vi "Receive Value Change Msg.vi"(8 "error in (no error)":errorcluster, 10 "ValueChangeMsg":refnum<class "ValueChangeMsg.lvclass">, 11 "MediatorBusMonitor In":refnum<class "MediatorBusMonitor.lvclass">) -> (0 "error out":errorcluster, 3 "MediatorBusMonitor Out":refnum<class "MediatorBusMonitor.lvclass">)   [LabVIEW 2015, in "Mediator.lvlib" / "MediatorBusMonitor.lvclass"]
doc: "<License>\nCopyright © 2017 Composed Systems, LLC | All rights reserved\nwww.composed.io\n\nAuthor: Ethan Stern <ethan.stern@composed.io>\n\nThis software is provided \"AS IS\" WITHOUT WARRANTIES, either express or implied, AND IS FOR EDUCATIONAL PURPOSES ONLY.\n</License>"
uses:
  MediatorBusMonitor.lvclass
  AutoRegistration/ActorAutoRegistration Messages/ValueChangeMsg/ValueChangeMsg.lvclass
  MediatorBusMonitor.lvclass/MediatorBusMonitor.ctl
  <vilib>/ActorFramework/Time-Delayed Send Message/Time-Delay Override Options.ctl
  MediatorBusMonitor Messages/Update Front Panel Msg/Update Front Panel Msg.lvclass
  <vilib>/ActorFramework/Actor/Actor.lvclass/Actor.ctl
  <vilib>/ActorFramework/Message Enqueuer/Message Enqueuer.lvclass/Message Enqueuer.ctl
  <vilib>/ActorFramework/Message Enqueuer/Init from Existing Queue.vi
  <vilib>/ActorFramework/Message Enqueuer/Message Enqueuer.lvclass
  Components/CurrentValueTable/CurrentValueTable.lvclass
  <vilib>/ActorFramework/Actor/Actor.lvclass
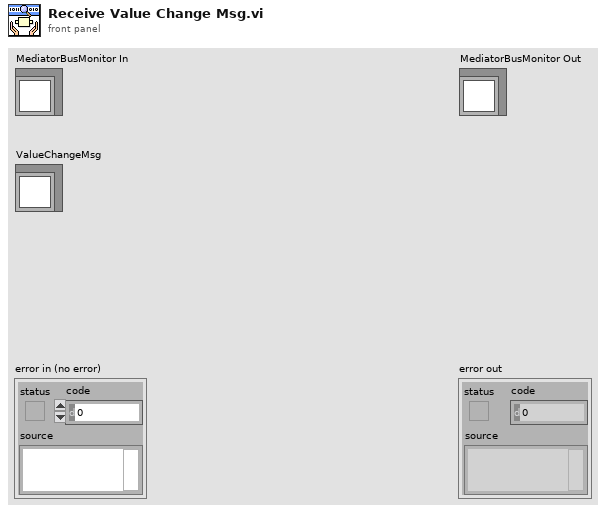
[diagram p1: front panel]
types:
  T1 = typedef "Time-Delay Override Options.ctl" = enum16{"Send next copy now", "Skip next scheduled copy", "Send next copy now and stop all further copies", "Stop all further copies"}
  T2 = typedef "CurrentValueTable.lvlib/CurrentValueTable.lvclass/CurrentValueTable Reference.ctl" = refnum<data-value>
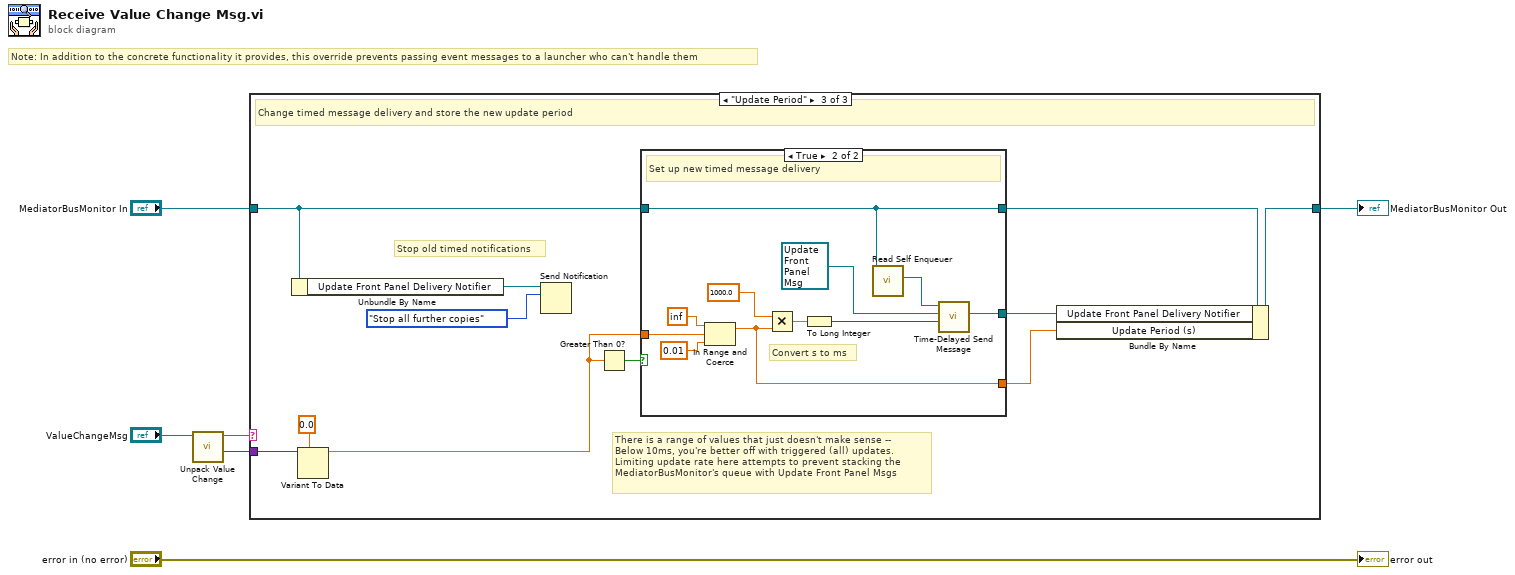
[diagram p0: block diagram]
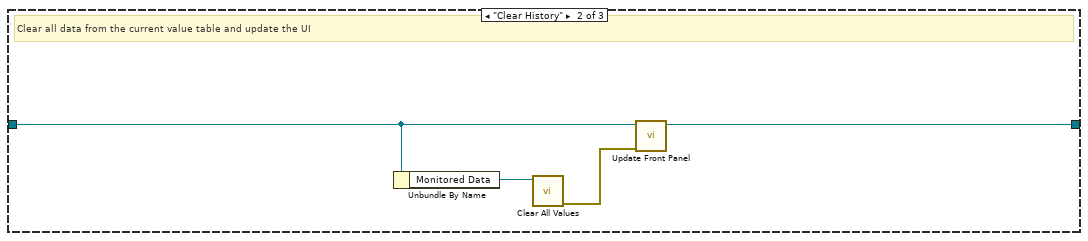
[diagram p3: hidden frame]
diagram:
  # "Note: In addition to the concrete functionality it provides, this override prevents passing event messages to a launcher who can't handle them"
  n1 = call-dynamic "Unpack Value Change.vi"("ValueChangeMsg In"="ValueChangeMsg") -> ("New Value"=w1:variant, "Name"=w4:string)  [unwired: 8 in, 1 out]
  n2 = case shown="\"Update Period\"" w4 {
    tunnel: "MediatorBusMonitor In" -> [w7 w11 w15]
    tunnel: [w7 w9 w22] -> w2
    tunnel: w1 -> [_ _ w21]
    frame Default {
      # "Do nothing by default"
    }
    frame "Clear History" {
      # "Clear all data from the current value table and update the UI"
      n3 = Unbundle By Name(w11) -> ("Monitored Data"=w10:T2)
      n4 = call "Clear All Values.vi"("Current Value Table"=w10) -> ("error out"=w8:errorcluster)  [unwired: 9 in, 1 out]
      n5 = call "Update Front Panel.vi"("error in (no error)"=w8, "MediatorBusMonitor In"=w11) -> ("MediatorBusMonitor Out"=w9:refnum<class "MediatorBusMonitor.lvclass">)  [unwired: 8 in, 1 out]
    }
    frame "Update Period" {
      # "There is a range of values that just doesn't make sense --\nBelow 10ms, you're better off with triggered (all) updates.\nLimiting update rate here attempts to prevent stacking the\nMediatorBusMonitor's queue with Update Front Panel Msgs"
      # "Stop old timed notifications"
      # "Change timed message delivery and store the new update period"
      n6 = Unbundle By Name(w15) -> ("Update Front Panel Delivery Notifier"=w14:refnum<notifier>)
      n7 = Variant To Data(type=0.0, Variant=w21) -> (data=w17:dbl)  [unwired: 1 in, 1 out]
      n8 = Send Notification(notification=Time-Delay_Override_Options."Stop all further copies", notifier=w14) -> ()  [unwired: 1 in, 2 out]
      n9 = Greater Than 0?(x=w17) -> (x > 0?=w16:bool)
      n10 = case shown="True" w16 {
        tunnel: w15 -> [w24 w30]
        tunnel: [_ w33] -> w19
        tunnel: w17 -> [w23 w26]
        tunnel: [w24 w30] -> w18
        tunnel: [w23 w25] -> w12
        frame False {
          # "No timed delivery (updates triggered by new data)"
        }
        frame True {
          # "Convert s to ms"
          # "Set up new timed message delivery"
          n11 = In Range and Coerce(upper limit=inf, x=w26, lower limit=0.01) -> (coerced(x)=w25:dbl)  [unwired: 1 out]
          n12 = Multiply(x=1000.0, y=w25) -> (x*y=w31:dbl)
          n13 = To Long Integer(number=w31) -> (32bit integer=w27:i32)
          n14 = call <vilib>:"Read Self Enqueuer.vi"("Actor"=w30) -> ("Self Enqueuer"=w34:refnum<class "Message Enqueuer.lvclass">)  [unwired: 10 in]
          n15 = call <vilib>:"Time-Delayed Send Message.vi"("Milliseconds To Wait"=w27, "Message"=refnum<class "Update Front Panel Msg.lvclass"> refnum ("Mediator.lvlib:Update Front Panel Msg.lvclass"), "Message Enqueuer"=w34) -> ("Delivery Notifier"=w33:refnum<notifier>)  [unwired: 7 in, 1 out]
        }
      }
      n16 = Bundle By Name(cluster=w18, "Update Front Panel Delivery Notifier"=w19, "Update Period (s)"=w12) -> (w22:refnum<class "MediatorBusMonitor.lvclass">)
    }
  }
  "MediatorBusMonitor Out" <- w2
  "error out" <- "error in (no error)"
